vi "SpecAn Configure AMPM.vi"(0 "RFmx Handle In":refnum<k21>, 1 "Selector String":string, 5 "RFmx SpecAn AMPM Configuration":T1={"Measurement Interval (s)"=0.0001, "DUT Average Input Power (dBm)"=-20.0, "Signal Type"=0, "Reference Waveform"={"Name"="Wfm", "Data"=refnum, "Signal Bandwidth (Hz)"=0.0, "PAPR (dB)"=0.0, "Burst Length (s)"=0.0, "Sample Rate"=0.0, "Burst Start Locations"=[], "Burst Stop Locations"=[], "Idle Duration Present?"=FALSE, "Runtime Scaling"=0.0, "Script"=""}} {"Reference Waveform"."Runtime Scaling" format="%#_6p"; "Reference Waveform"."Sample Rate" format="%#_6p"; "Reference Waveform"."Burst Length (s)" format="%#_6p"; "Reference Waveform"."PAPR (dB)" format="%.2f"; "Reference Waveform"."Signal Bandwidth (Hz)" format="%#_6p"; "Signal Type" items=["Modulated", "Tones"]; "DUT Average Input Power (dBm)" format="%.2f"; "Measurement Interval (s)" format="%.2p"}, 11 "error in (no error)":errorcluster) -> (4 "RFmx Handle Out":refnum<k21>, 15 "error out":errorcluster)   [LabVIEW 2016, in "RFmxSpecAn.lvlib"]
uses:
  RFmxSpecAn.lvlib
  Typedefs/SpecAn AMPM Configuration.ctl
  SG/Typedefs/Waveform.ctl
  <resource>/objmgr/RFmxSpecAn.rc
  SG/SG.lvlib
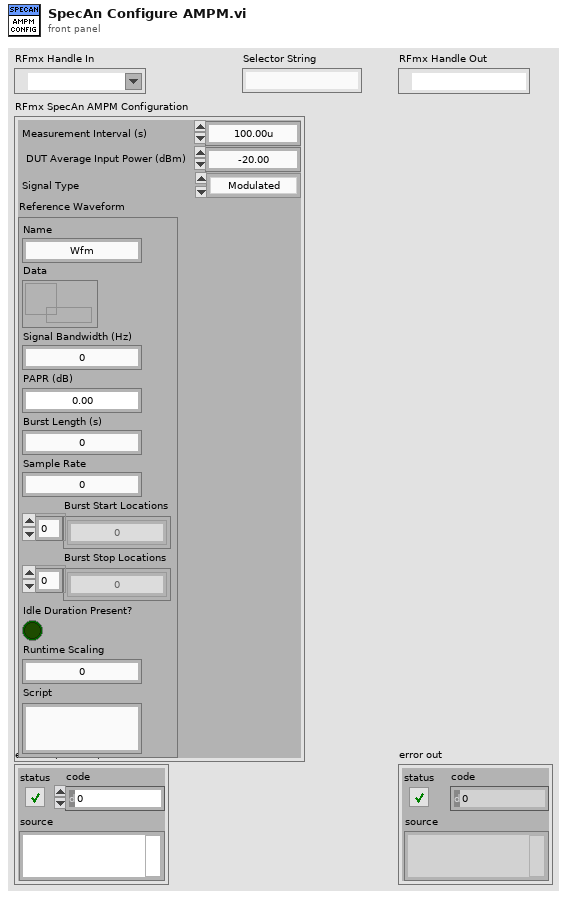
[diagram p1: front panel]
types:
  T1 = typedef "RFmxSpecAn.lvlib/SpecAn AMPM Configuration.ctl" = cluster{"Measurement Interval (s)":dbl, "DUT Average Input Power (dBm)":dbl, "Signal Type":i32, "Reference Waveform":T2}
  T2 = typedef "SG.lvlib/Waveform.ctl" = cluster{"Name":string, "Data":refnum<data-value>, "Signal Bandwidth (Hz)":dbl, "PAPR (dB)":dbl, "Burst Length (s)":dbl, "Sample Rate":dbl, "Burst Start Locations":i32[], "Burst Stop Locations":i32[], "Idle Duration Present?":bool, "Runtime Scaling":dbl, "Script":string}
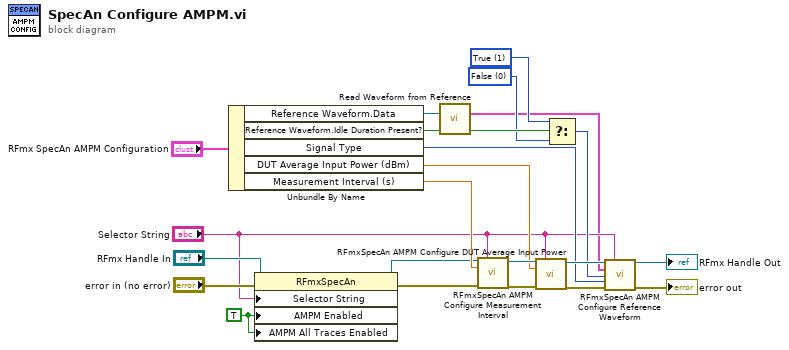
[diagram p0: block diagram]
diagram:
  w7 = 0 items=["False", "True"] ("Idle Duration Present")
  w10 = 1 items=["False", "True"] ("Idle Duration Present")
  w12 = TRUE ("AMPM Enabled")
  n1 = Unbundle By Name("RFmx SpecAn AMPM Configuration") -> ("Reference Waveform.Data"=w22:refnum<data-value>, "Reference Waveform.Idle Duration Present?"=w8:bool, "Signal Type"=w11:i32, "DUT Average Input Power (dBm)"=w6:dbl, "Measurement Interval (s)"=w5:dbl)
  n2 = property class="RFmxSpecAn"(reference="RFmx Handle In", error in="error in (no error)", "Selector String"="Selector String", "AMPM Enabled"=w12, "AMPM All Traces Enabled"=w12) -> (reference out=w4:refnum<k21>, error out=w13:errorcluster)
  n3 = call "Read Waveform from Reference.vi"("Data"=w22) -> ("Waveform"=w1:cluster{"t0":dbl, "dt":dbl, "y":csg[]})  [unwired: 13 in, 1 out]
  n4 = call <vilib>:"RFmxSpecAn AMPM Configure Measurement Interval.vi"("Instrument Handle In"=w4, "Selector String"="Selector String", "Measurement Interval (s)"=w5, "error in (no error)"=w13) -> ("Instrument Handle Out"=w21:refnum<k21>, "error out"=w20:errorcluster)  [unwired: 10 in]
  n5 = call <vilib>:"RFmxSpecAn AMPM Configure DUT Average Input Power.vi"("Instrument Handle In"=w21, "Selector String"="Selector String", "DUT Average Input Power (dBm)"=w6, "error in (no error)"=w20) -> ("Instrument Handle Out"=w19:refnum<k21>, "error out"=w18:errorcluster)  [unwired: 10 in]
  n6 = Select(t=w10, s=w8, f=w7) -> (s? t:f=w9:i32)
  n7 = call <vilib>:"RFmxSpecAn AMPM Configure Reference Waveform.vi"("Instrument Handle In"=w19, "Selector String"="Selector String", "Reference Waveform"=w1, "Idle Duration Present"=w9, "Signal Type"=w11, "error in (no error)"=w18) -> ("Instrument Handle Out"=→"RFmx Handle Out":refnum<k21>, "error out"=→"error out":errorcluster)  [unwired: 8 in]
